vi "Union Msgs.vi"(9 "Msgs":T1, 10 "Msgs":T1[](array[typedef])) -> (2 "Union of Msgs":T1)   [LabVIEW 2025, in "jettl.lvlib"]
uses:
  jettl.lvlib
  Msgs.ctl
  Msg/Msg.lvclass
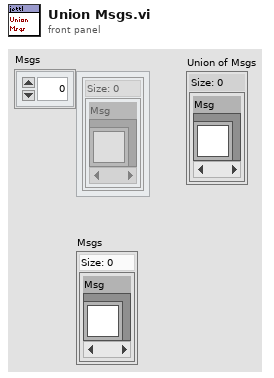
[diagram p1: front panel]
types:
  T1 = typedef "jettl.lvlib/Msgs.ctl" = set{refnum<class "Msg.lvclass">}
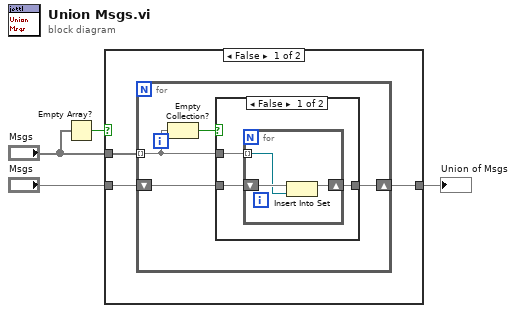
[diagram p0: block diagram]
diagram:
  n1 = Empty Array?(array="Msgs") -> (empty?=w4:bool)
  n2 = case shown="False" w4 {
    tunnel: "Msgs" -> [w7 _]
    tunnel: "Msgs" -> [w6 w19]
    tunnel: [w5 w19] -> w2
    frame False {
      n3 = for {
        tunnel: w7 -> [w9] mode=indexing
        shift-right: [w10] -> w5
        shift-left: w6 -> [w11]
        n4 = Empty Collection?(1:w9) -> (0:w8:bool)
        n5 = case shown="False" w8 {
          tunnel: w11 -> [w14 w18]
          tunnel: [w13 w18] -> w10
          tunnel: w9 -> [w12 _]
          frame False {
            n6 = for {
              shift-right: [w16] -> w13
              shift-left: w14 -> [w17]
              tunnel: w12 -> [w15] mode=indexing
              n7 = Insert Into Set(10:w15, 11:w17) -> (3:w16:T1)  [unwired: 1 out]
            }
          }
          frame True {
          }
        }
      }
    }
    frame True {
    }
  }
  "Union of Msgs" <- w2
